vi "Get Request Type.vi"(8 "error in (no error)":errorcluster, 11 "GetHotkeyList in":refnum<class "GetHotkeyList.lvclass">) -> (0 "error out":errorcluster, 2 "Request Type":string, 3 "GetHotkeyList out":refnum<class "GetHotkeyList.lvclass">)   [LabVIEW 2022 SP3, in "obs-websocket-lv.lvlib" / "GetHotkeyList.lvclass"]
uses:
  GetHotkeyList.lvclass
  GetHotkeyList.lvclass/GetHotkeyList.ctl
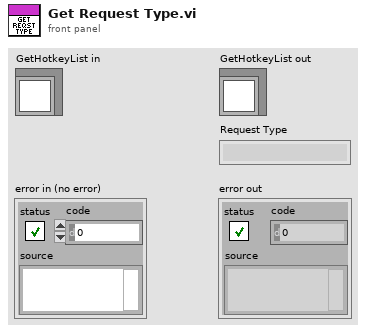
[diagram p1: front panel]
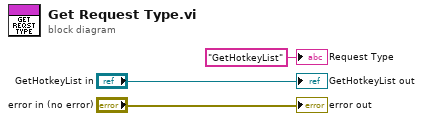
[diagram p0: block diagram]
diagram:
  "error out" <- "error in (no error)"
  "GetHotkeyList out" <- "GetHotkeyList in"
  "Request Type" <- "GetHotkeyList" ("Request Type")
